vi "saveTestParameters.vi"(8 "error in (no error)":errorcluster, 11 "Logger in":refnum<class "TestDataLog.lvclass">) -> (0 "error out":errorcluster, 3 "Logger out":refnum<class "TestDataLog.lvclass">)   [LabVIEW 2013, in "TestDataLog.lvclass"]
uses:
  TestDataLog.lvclass
  <userlib>/Common/Log/Log/Log.lvclass/Log.ctl
  TestDataLog.lvclass/TestDataLog.ctl
  <userlib>/Common/Log/Log/Log.lvclass
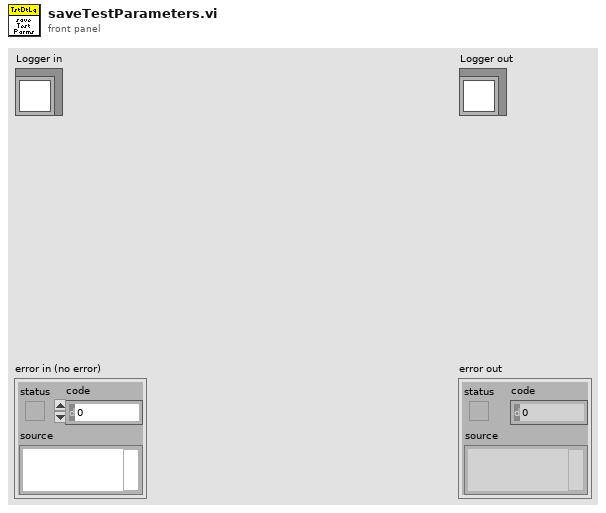
[diagram p1: front panel]
types:
  T1 = typedef "TestParameters.ctl" = cluster{"Number of cycles for complete test":u32, "Cycle profile":T2}
  T2 = typedef "CycleProfileConfig.ctl" = cluster{"Force Setpoint":dbl[unit][], "Pause After":dbl[unit][]}
  T3 = typedef "SystemController.ctl" = cluster{"PID Gains":T4, "Force Error In Range Limit":dbl[unit]}
  T4 = typedef "PIDGains.ctl" = cluster{"Proportional Gain (Kc)":dbl, "Integral Time (Ti, min)":dbl, "Derivative Time (Td, min)":dbl}
  T5 = typedef "Log.lvlib/Log.ctl" = cluster{"Log Directory":path, "Log Filename Base":string, "Max records per file":u32, "Comment":string}
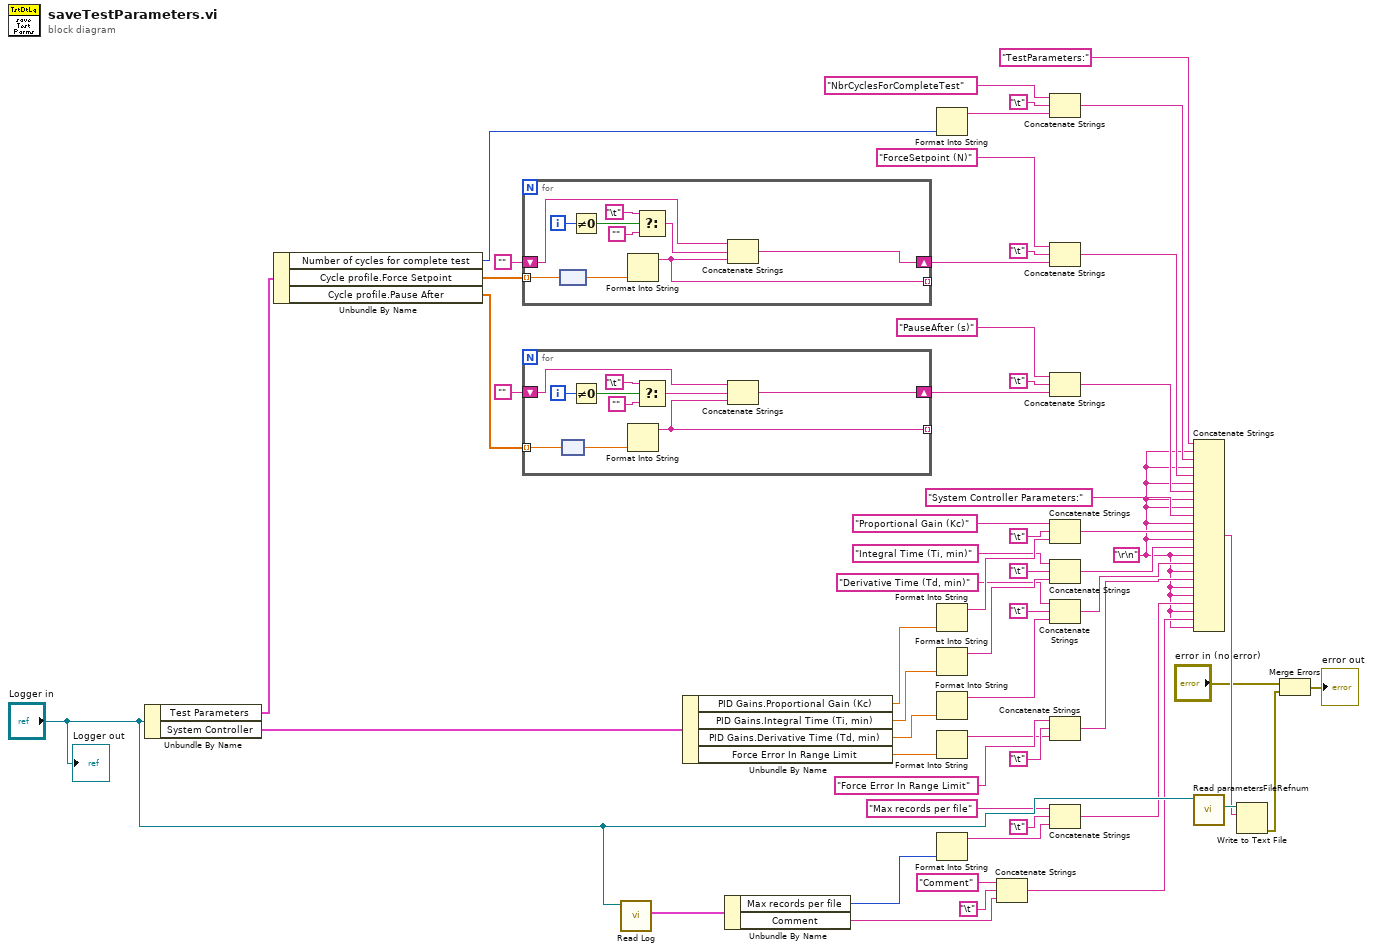
[diagram p0: block diagram]
diagram:
  w6 = "\r\n"
  n1 = Unbundle By Name("Logger in") -> ("Test Parameters"=w58:T1, "System Controller"=w52:T3)
  n2 = Unbundle By Name(w58) -> ("Number of cycles for complete test"=w57:u32, "Cycle profile.Force Setpoint"=w56:dbl[unit][], "Cycle profile.Pause After"=w54:dbl[unit][])
  n3 = for {
    tunnel: w56 -> [w63] mode=indexing
    shift-right: [w68] -> w37
    shift-left: "" -> [w67]
    tunnel: [w64] -> _ mode=indexing
    i -> [w66]
    n4 = node(w63) -> (w62:dbl)
    n5 = Not Equal To 0?(x=w66) -> (x != 0?=w65:bool)
    n6 = Format Into String(w62) -> (resulting string=w64:string)  [unwired: 3 in, 1 out]
    n7 = Select(t="\t", s=w65, f="") -> (s? t:f=w59:string)
    n8 = Concatenate Strings(w67, w59, w64) -> (w68:string)
  }
  n9 = for {
    tunnel: w54 -> [w73] mode=indexing
    shift-right: [w78] -> w33
    shift-left: "" -> [w77]
    tunnel: [w74] -> _ mode=indexing
    i -> [w76]
    n10 = node(w73) -> (w72:dbl)
    n11 = Not Equal To 0?(x=w76) -> (x != 0?=w75:bool)
    n12 = Format Into String(w72) -> (resulting string=w74:string)  [unwired: 3 in, 1 out]
    n13 = Select(t="\t", s=w75, f="") -> (s? t:f=w69:string)
    n14 = Concatenate Strings(w77, w69, w74) -> (w78:string)
  }
  n15 = call <userlib>:"Read Log.vi"("Log in"="Logger in") -> ("Log"=w47:T5)  [unwired: 9 in, 1 out]
  n16 = Unbundle By Name(w52) -> ("PID Gains.Proportional Gain (Kc)"=w51:dbl, "PID Gains.Integral Time (Ti, min)"=w50:dbl, "PID Gains.Derivative Time (Td, min)"=w49:dbl, "Force Error In Range Limit"=w48:dbl[unit])
  n17 = Unbundle By Name(w47) -> ("Max records per file"=w46:u32, "Comment"=w9:string)
  n18 = Format Into String(w57) -> (resulting string=w40:string)  [unwired: 3 in, 1 out]
  n19 = Format Into String(w51) -> (resulting string=w25:string)  [unwired: 3 in, 1 out]
  n20 = Format Into String(w50) -> (resulting string=w23:string)  [unwired: 3 in, 1 out]
  n21 = Format Into String(w49) -> (resulting string=w21:string)  [unwired: 3 in, 1 out]
  n22 = Format Into String(w48) -> (resulting string=w19:string)  [unwired: 3 in, 1 out]
  n23 = Format Into String(w46) -> (resulting string=w11:string)  [unwired: 3 in, 1 out]
  n24 = Concatenate Strings("Comment" ("element"), "\t", w9) -> (w7:string)
  n25 = Concatenate Strings("NbrCyclesForCompleteTest" ("element"), "\t", w40) -> (w42:string)
  n26 = Concatenate Strings("ForceSetpoint (N)" ("element"), "\t", w37) -> (w36:string)
  n27 = Concatenate Strings("PauseAfter (s)" ("element"), "\t", w33) -> (w32:string)
  n28 = Concatenate Strings("Proportional Gain (Kc)" ("element"), "\t", w25) -> (w18:string)
  n29 = Concatenate Strings("Integral Time (Ti, min)" ("element"), "\t", w23) -> (w17:string)
  n30 = Concatenate Strings("Derivative Time (Td, min)" ("element"), "\t", w21) -> (w16:string)
  n31 = Concatenate Strings("Force Error In Range Limit" ("element"), "\t", w19) -> (w15:string)
  n32 = Concatenate Strings("Max records per file" ("element"), "\t", w11) -> (w8:string)
  n33 = Concatenate Strings("TestParameters:", w6, w42, w6, w36, w6, w32, w6, w6, "System Controller Parameters:" ("element"), w6, w18, w6, w17, w6, w16, w6, w15, w6, w6, w8, w6, w7, w6) -> (w4:string)
  n34 = call <userlib>:"Read parametersFileRefnum.vi"("Log in"="Logger in") -> ("parametersFileRefnum"=w5:refnum<file>)  [unwired: 9 in, 1 out]
  n35 = Write to Text File(file (use dialog)=w5, text=w4) -> (error out=w2:errorcluster)  [unwired: 2 in, 2 out]
  n36 = Merge Errors("error in (no error)", w2) -> (→"error out":errorcluster)
  "Logger out" <- "Logger in"
